vi "initialize vi references.vi"(7 "runtime class path":path, 8 "error in":errorcluster, 9 "output in":T4, 10 "process in":T5, 11 "input in":T3) -> (0 "error out":errorcluster, 3 "initialized references":T1[](array[typedef]))   [LabVIEW 2013]
uses:
  processing script control.ctl
  output script control.ctl
  input script control.ctl
  initialized references.ctl
  interface VI type.ctl
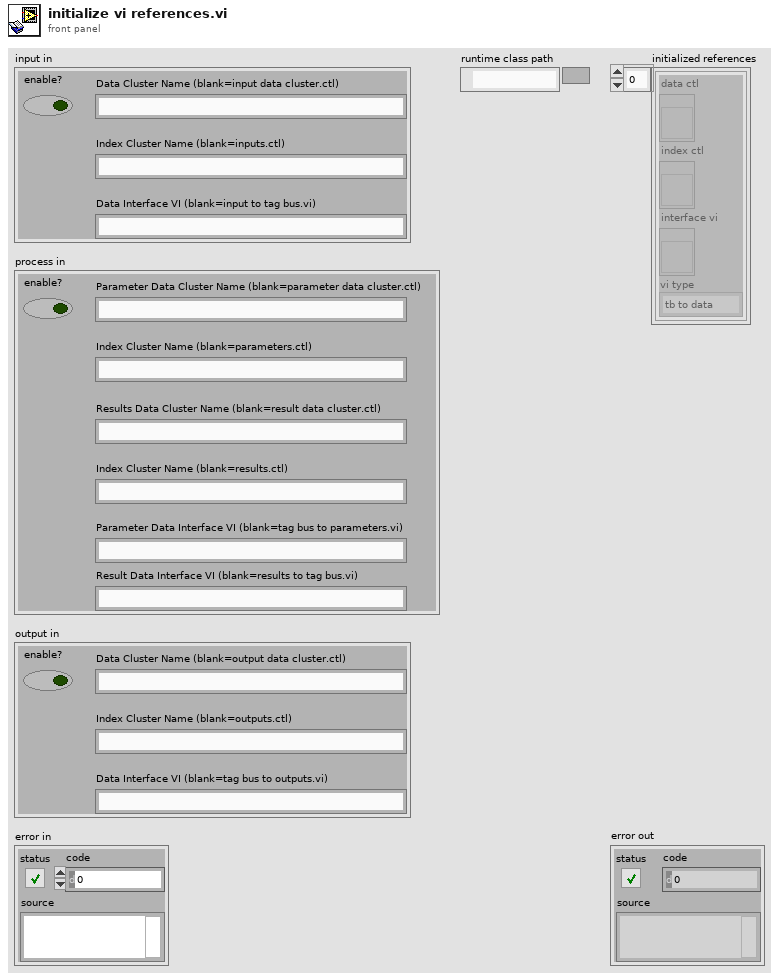
[diagram p1: front panel]
types:
  T1 = typedef "initialized references.ctl" = cluster{"data ctl":refnum<vi>, "index ctl":refnum<vi>, "interface vi":refnum<vi>, "vi type":T2}
  T2 = typedef "interface VI type.ctl" = enum16{"tb to data", "data to tb"}
  T3 = typedef "input script control.ctl" = cluster{"enable?":bool, "Data Cluster Name (blank=input data cluster.ctl)":string, "Index Cluster Name (blank=inputs.ctl)":string, "Data Interface VI (blank=input to tag bus.vi)":string}
  T4 = typedef "output script control.ctl" = cluster{"enable?":bool, "Data Cluster Name (blank=output data cluster.ctl)":string, "Index Cluster Name (blank=outputs.ctl)":string, "Data Interface VI (blank=tag bus to outputs.vi)":string}
  T5 = typedef "processing script control.ctl" = cluster{"enable?":bool, "Parameter Data Cluster Name (blank=parameter data cluster.ctl)":string, "Index Cluster Name (blank=parameters.ctl)":string, "Results Data Cluster Name (blank=result data cluster.ctl)":string, "Index Cluster Name (blank=results.ctl)":string, "Parameter Data Interface VI (blank=tag bus to parameters.vi)":string, "Result Data Interface VI (blank=results to tag bus.vi)":string}
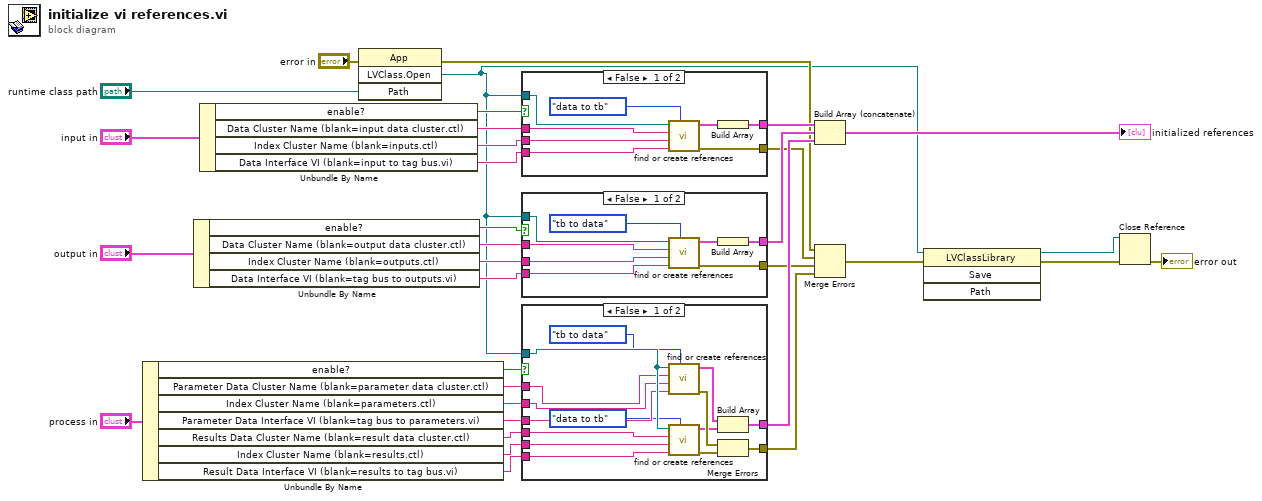
[diagram p0: block diagram]
diagram:
  n1 = Unbundle By Name("process in") -> ("enable?"=w24:bool, "Parameter Data Cluster Name (blank=parameter data cluster.ctl)"=w23:string, "Index Cluster Name (blank=parameters.ctl)"=w22:string, "Parameter Data Interface VI (blank=tag bus to parameters.vi)"=w21:string, "Results Data Cluster Name (blank=result data cluster.ctl)"=w16:string, "Index Cluster Name (blank=results.ctl)"=w17:string, "Result Data Interface VI (blank=results to tag bus.vi)"=w18:string)
  n2 = Unbundle By Name("output in") -> ("enable?"=w25:bool, "Data Cluster Name (blank=output data cluster.ctl)"=w26:string, "Index Cluster Name (blank=outputs.ctl)"=w27:string, "Data Interface VI (blank=tag bus to outputs.vi)"=w28:string)
  n3 = Unbundle By Name("input in") -> ("enable?"=w32:bool, "Data Cluster Name (blank=input data cluster.ctl)"=w31:string, "Index Cluster Name (blank=inputs.ctl)"=w30:string, "Data Interface VI (blank=input to tag bus.vi)"=w29:string)
  n4 = invoke class="App" method="LVClass.Open"(error in="error in", "Path"="runtime class path") -> (error out=w5:errorcluster, "LVClass.Open"=w2:refnum<vi>)  [unwired: 2 in, 2 out]
  n5 = case shown="False" w32 {
    tunnel: w31 -> [w41 _]
    tunnel: w30 -> [w39 _]
    tunnel: w29 -> [w38 _]
    tunnel: w2 -> [w40 _]
    tunnel: [w36 _] -> w14
    tunnel: [w35 _] -> w7
    frame False {
      n6 = call "find or create references.vi"("vi type"=interface_VI_type."data to tb", "Data Interface VI"=w38, "Index Cluster Name"=w39, "Data Cluster Name"=w41, "LVClassLibrary in"=w40) -> ("error out"=w35:errorcluster, "vi refs"=w37:T1)  [unwired: 5 in]
      n7 = Build Array(w37) -> (w36:T1[])
    }
    frame True {
    }
  }
  n8 = case shown="False" w25 {
    tunnel: w26 -> [w46 _]
    tunnel: w27 -> [w45 _]
    tunnel: w28 -> [w44 _]
    tunnel: [w48 _] -> w13
    tunnel: w2 -> [w47 _]
    tunnel: [w43 _] -> w6
    frame False {
      n9 = call "find or create references.vi"("vi type"=interface_VI_type."tb to data", "Data Interface VI"=w44, "Index Cluster Name"=w45, "Data Cluster Name"=w46, "LVClassLibrary in"=w47) -> ("error out"=w43:errorcluster, "vi refs"=w49:T1)  [unwired: 5 in]
      n10 = Build Array(w49) -> (w48:T1[])
    }
    frame True {
    }
  }
  n11 = case shown="False" w24 {
    tunnel: w23 -> [w52 _]
    tunnel: w22 -> [w53 _]
    tunnel: w21 -> [w54 _]
    tunnel: w18 -> [w57 _]
    tunnel: w17 -> [w56 _]
    tunnel: w16 -> [w55 _]
    tunnel: [w63 _] -> w10
    tunnel: [w59 _] -> w8
    tunnel: w2 -> [w58 _]
    frame False {
      n12 = call "find or create references.vi"("vi type"=interface_VI_type."tb to data", "Data Interface VI"=w54, "Index Cluster Name"=w53, "Data Cluster Name"=w52, "LVClassLibrary in"=w58) -> ("error out"=w62:errorcluster, "vi refs"=w64:T1)  [unwired: 5 in]
      n13 = call "find or create references.vi"("vi type"=interface_VI_type."data to tb", "Data Interface VI"=w57, "Index Cluster Name"=w56, "Data Cluster Name"=w55, "LVClassLibrary in"=w58) -> ("error out"=w61:errorcluster, "vi refs"=w60:T1)  [unwired: 5 in]
      n14 = Build Array(w64, w60) -> (w63:T1[])
      n15 = Merge Errors(w62, w61) -> (w59:errorcluster)
    }
    frame True {
    }
  }
  n16 = Build Array (concatenate)(w14, w13, w10) -> (→"initialized references":T1[])
  n17 = Merge Errors(w5, w7, w6, w8) -> (w11:errorcluster)
  n18 = invoke class="LVClassLibrary" method="Save"(reference=w2, error in=w11) -> (reference out=w1:refnum<vi>, error out=w3:errorcluster)  [unwired: 2 in, 2 out]
  n19 = Close Reference(reference=w1, error in (no error)=w3) -> (error out=→"error out":errorcluster)
